vi "Command Dispatch.vi"(8 "error in (no error)":errorcluster, 10 "GUID-cmd-data":T1, 11 "Controller in":refnum<class "Controller.lvclass">) -> (0 "error out":errorcluster, 3 "Controller out":refnum<class "Controller.lvclass">)   [LabVIEW 2016, in "Controller Actor.lvlib" / "Controller.lvclass"]
uses:
  <userlib>/Common Components/Controller/Controller.lvclass
  <userlib>/Common Components/Common/GUID-command-data.ctl
  <userlib>/Common Components/Function Messages/Command Dispatch Msg/Command Dispatch Msg.lvclass/Command Dispatch Msg.ctl
  <vilib>/ActorFramework/Message Enqueuer/Message Enqueuer.lvclass/Message Enqueuer.ctl
  <vilib>/ActorFramework/Message Enqueuer/Enqueue.vi
  <userlib>/Common Components/Function Messages/Command Dispatch Msg/Command Dispatch Msg.lvclass
  C:/Program Files (x86)/National Instruments/LabVIEW 2016/vi.lib/ActorFramework/Message/Message.lvclass
  <vilib>/ActorFramework/Message Priority Queue/Priority Enqueue.vi
  <userlib>/Common Components/Common/Common.lvlib
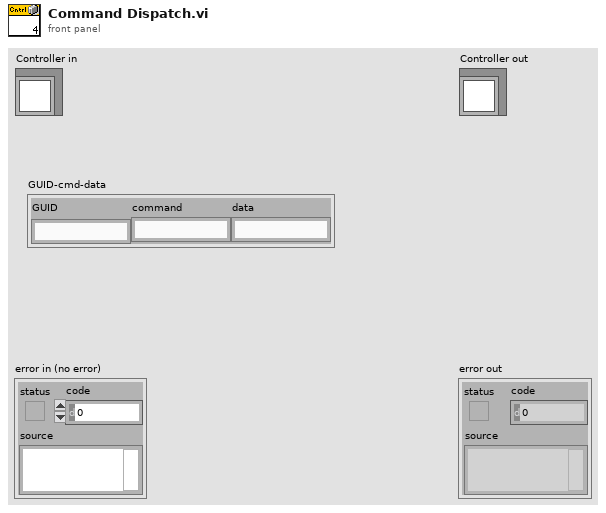
[diagram p1: front panel]
types:
  T1 = typedef "Common.lvlib/GUID-command-data.ctl" = cluster{"GUID":string, "command":string, "data":string}
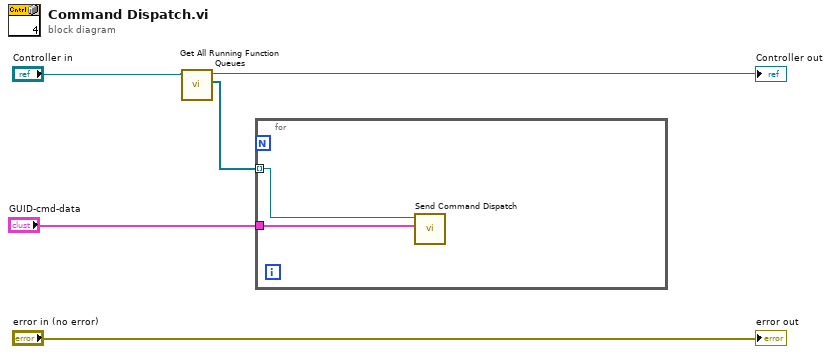
[diagram p0: block diagram]
diagram:
  n1 = call <userlib>:"Get All Running Function Queues.vi"("Controller in"="Controller in") -> ("Array of Function Queues"=w2:refnum<class "Message Enqueuer.lvclass">[], "Controller out"=→"Controller out":refnum<class "Controller.lvclass">)  [unwired: 8 in, 1 out]
  n2 = for {
    tunnel: w2 -> [w7] mode=indexing
    tunnel: "GUID-cmd-data" -> [w6]
    n3 = call <userlib>:"Send Command Dispatch.vi"("GUID-cmd-data"=w6, "Message Enqueuer"=w7) -> ()  [unwired: 8 in, 2 out]
  }
  "error out" <- "error in (no error)"
